vi "sendSingle.vi"(0 "refer":refnum<queue>, 1 "to":string, 2 "from":string, 3 "data":variant, 4 "priority":bool, 5 "errorIn":errorcluster, 6 "remark1":string, 7 "index":i32, 8 "remark 2":string) -> (14 "refer":refnum<queue>, 19 "errorOut":errorcluster)   [LabVIEW 2017]
uses:
  models/EMSGData.ctl
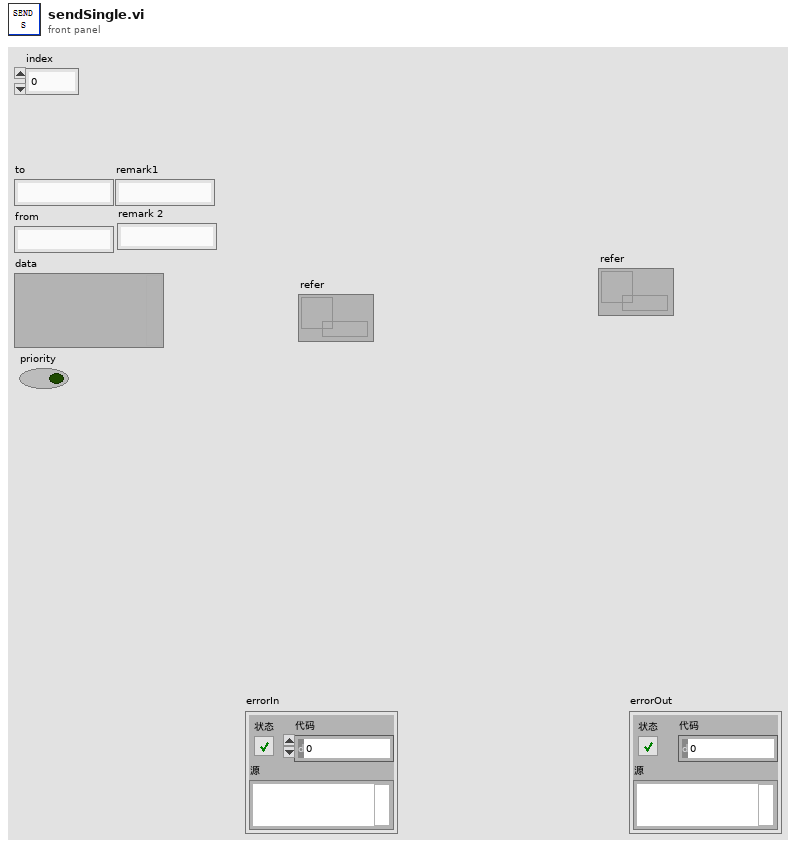
[diagram p1: front panel]
types:
  T1 = typedef "EMSGData.ctl" = cluster{"to":string, "from":string, "data":variant, "remark1":string, "remark 2":string}
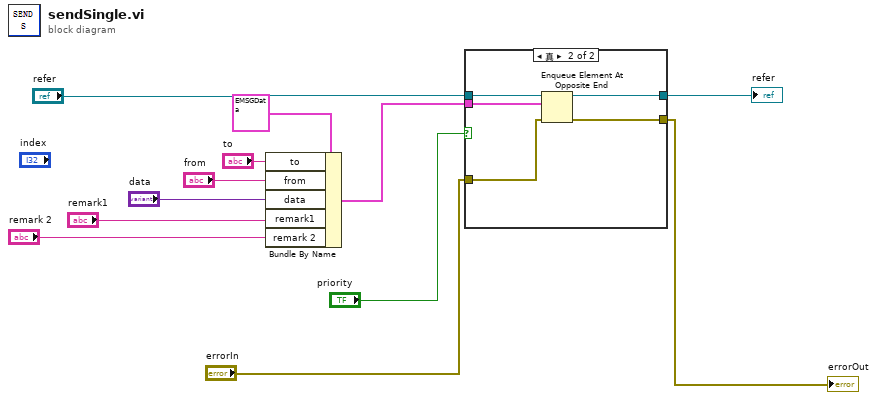
[diagram p0: block diagram]
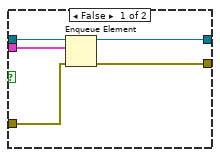
[diagram p2: hidden frame]
diagram:
  n1 = Bundle By Name(cluster=T1 {"to"="", "from"="", "data"=variant, "remark1"="", "remark 2"=""} ("EMSGData"), "to"="to", "from"="from", "data"="data", "remark1"="remark1", "remark 2"="remark 2") -> (w5:T1)
  n2 = case shown="真" "priority" {
    tunnel: "refer" -> [w17 w22]
    tunnel: w5 -> [w16 w21]
    tunnel: "errorIn" -> [w15 w20]
    tunnel: [w14 w19] -> w2
    tunnel: [w13 w18] -> w1
    frame False {
      n3 = Enqueue Element(queue=w17, element=w16, error in (no error)=w15) -> (queue out=w13:refnum<queue>, error out=w14:errorcluster)  [unwired: 1 in, 1 out]
    }
    frame True {
      n4 = Enqueue Element At Opposite End(queue=w22, element=w21, error in (no error)=w20) -> (queue out=w18:refnum<queue>, error out=w19:errorcluster)  [unwired: 1 in, 1 out]
    }
  }
  "errorOut" <- w2
  "refer" <- w1
